vi "Consumer.vi"(8 "error in (no error)":errorcluster, 9 "Data":variant, 10 "Case ID":string, 11 "uService Template in":refnum<class "Template Internal uService.lvclass">) -> (0 "error out":errorcluster, 3 "uService Template out":refnum<class "Template Internal uService.lvclass">)   [LabVIEW 2026, in "TALOS.lvlib" / "Template Internal uService.lvlib" / "Template Internal uService.lvclass"]
uses:
  Template Internal uService.lvclass
  Template Internal uService Consumer Case Selector.ctl
  Father of all uServices/Father of all uServices/Father of all uServices.lvclass
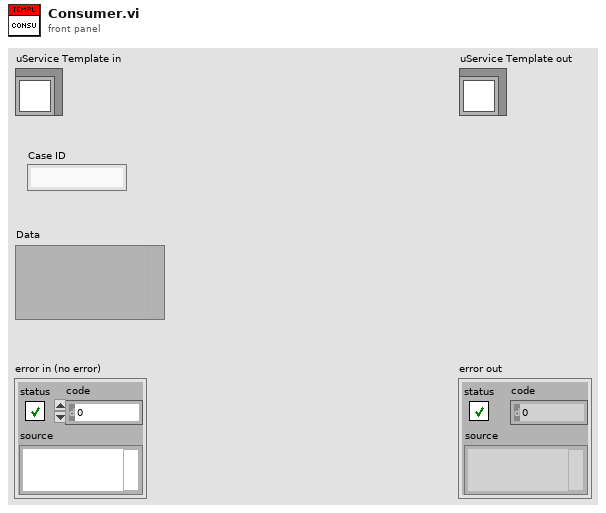
[diagram p1: front panel]
types:
  T1 = typedef "TALOS.lvlib/Template Internal uService.lvlib/Template Internal uService.lvclass/Template Internal uService Consumer Case Selector.ctl" = enum16{"Example"}
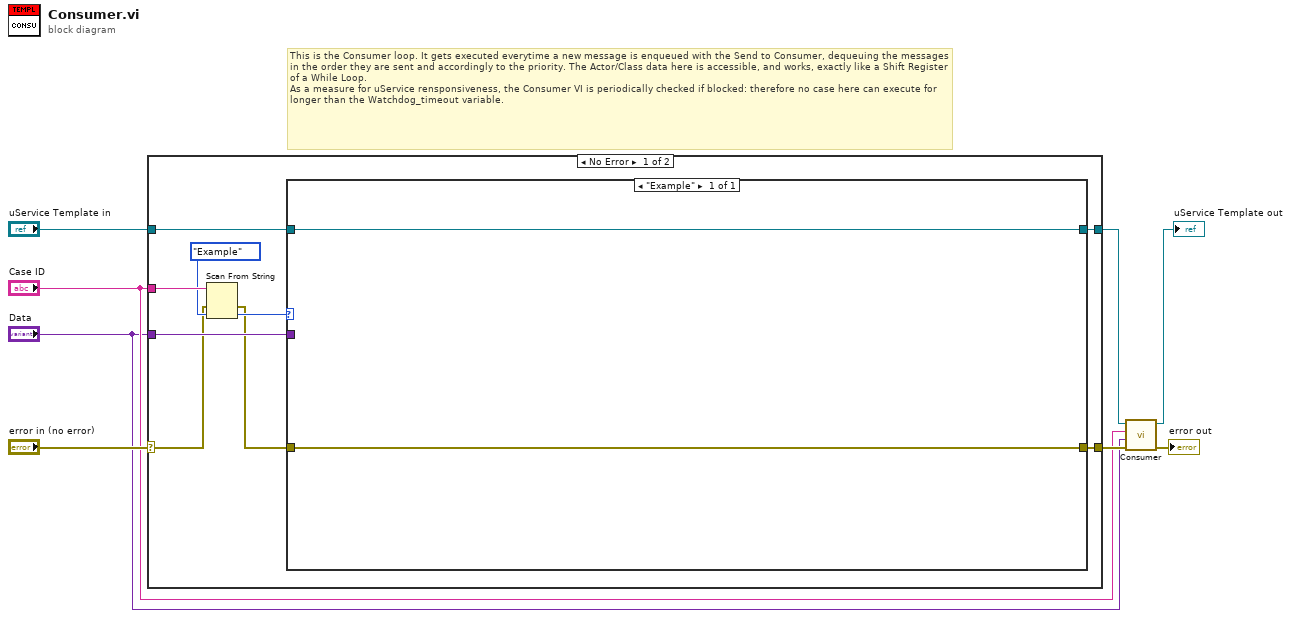
[diagram p0: block diagram]
diagram:
  # "This is the Consumer loop. It gets executed everytime a new message is enqueued with the Send to Consumer, dequeuing the messages in the order they are sent and accordingly to the priority. The Actor/Class data here is accessible, and works, exactly like a Shift Register of a While Loop. \nAs a measure for uService rensponsiveness, the Consumer VI is periodically checked if blocked: therefore no case here can execute for longer than the Watchdog_timeout variable."
  n1 = case shown="No Error" "error in (no error)" {
    selector: "error in (no error)" -> [w10 w20]
    tunnel: "uService Template in" -> [w16 w21]
    tunnel: [w14 w21] -> w4
    tunnel: [w15 w20] -> w3
    tunnel: "Case ID" -> [w13 _]
    tunnel: "Data" -> [w17 _]
    frame No Error {
      n2 = Scan From String(input string=w13, error in=w10, default 1=Template_Internal_uService_Consumer_Case_Selector."Example") -> (error out=w9:errorcluster, output 1=w11:T1)  [unwired: 2 in, 2 out]
      n3 = case shown="\"Example\"" w11 {
        tunnel: w17 -> [_]
        tunnel: w9 -> [w18]
        tunnel: w16 -> [w19]
        tunnel: [w18] -> w15
        tunnel: [w19] -> w14
        frame "Example" {
        }
      }
    }
    frame Error {
    }
  }
  n4 = call-parent "Consumer.vi"("error in (no error)"=w3, "Data"="Data", "Case ID"="Case ID", "uService Template in"=w4) -> ("error out"=→"error out":errorcluster, "uService Template out"=→"uService Template out":refnum<class "Template Internal uService.lvclass">)  [unwired: 6 in]
